vi "Calc_Checksum.vi"(11 "DataFrame":u8[](array[numeric]) format="%04x") -> (3 "Checksum":u8 format="%b")   [LabVIEW 2019]
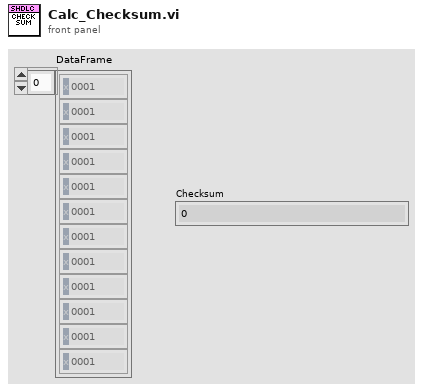
[diagram p1: front panel]
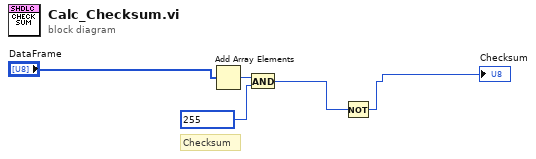
[diagram p0: block diagram]
diagram:
  # "Checksum"
  n1 = Add Array Elements(numeric array="DataFrame") -> (sum=w4:u8)
  n2 = And(x=w4, y=u8 255) -> (x .and. y?=w2:u8)
  n3 = Not(x=w2) -> (.not. x?=→"Checksum":u8)
